vi "XML_EEG_MatLabStringToWaveform.vi"(8 "error in (no error)":errorcluster, 9 "SampleRateHz":dbl, 11 "Hex String in":string) -> (0 "error out":errorcluster, 3 "Waveform out":waveform(dbl))   [LabVIEW 2016, in "XML_EEG_File_Parser.lvlib"]
uses:
  XML_EEG_File_Parser.lvlib
panel:
  # "This VI is a part of BCI Design library, http://www.ru-bci.org \nCopyright © 2020, Sotnikov Peter, All rights reserved. License: GNU GPLv3"
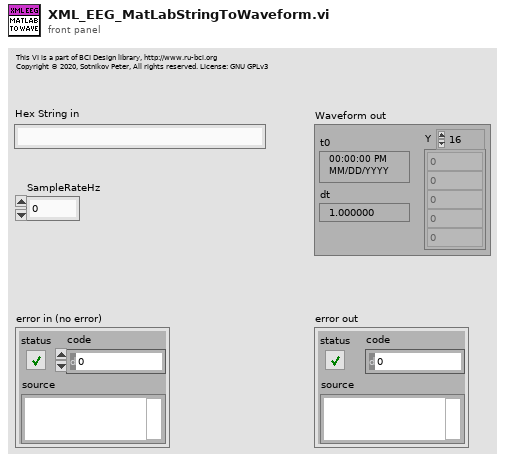
[diagram p1: front panel]
types:
  T1 = enum16{"big-endian, network order", "native, host order", "little-endian"}
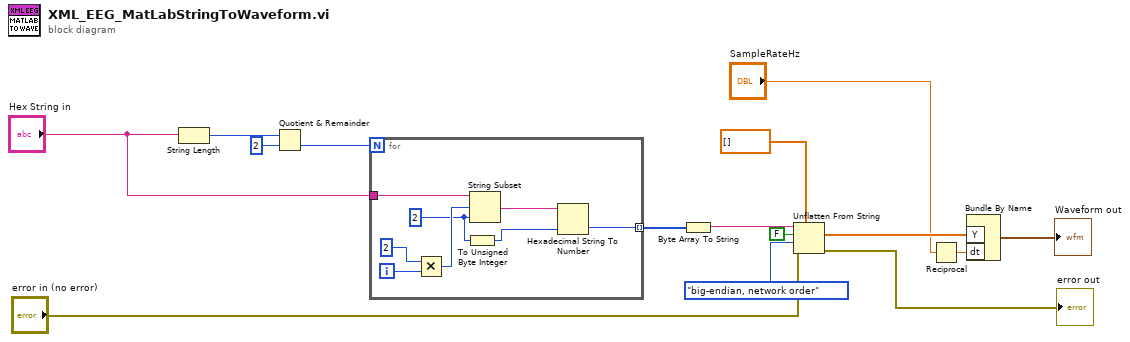
[diagram p0: block diagram]
diagram:
  n1 = String Length(string="Hex String in") -> (length=w15:i32)
  n2 = Quotient & Remainder(x=w15, y=2) -> (floor(x/y)=w13:i32)  [unwired: 1 out]
  n3 = for {
    N: w13 -> [_]
    tunnel: "Hex String in" -> [w23]
    tunnel: [w16] -> w11 mode=indexing
    i -> [w22]
    w18 = 2 ("length (rest)")
    n4 = Multiply(x=2, y=w22) -> (x*y=w20:i32)
    n5 = To Unsigned Byte Integer(number=w18) -> (unsigned 8bit integer=w19:u8)
    n6 = String Subset(string=w23, offset (0)=w20, length (rest)=w18) -> (substring=w17:string)
    n7 = Hexadecimal String To Number(string=w17, default (0uL)=w19) -> (number=w16:u8)  [unwired: 1 in, 1 out]
  }
  n8 = Byte Array To String(unsigned byte array=w11) -> (string=w10:string)
  n9 = Unflatten From String(type=dbl[] [], binary string=w10, data includes array or string size? (T)=FALSE, byte order (0:big-endian, network order)=T1."big-endian, network order", error in (no error)="error in (no error)") -> (value=w3:dbl[], error out=→"error out":errorcluster)  [unwired: 1 out]
  n10 = Reciprocal(x="SampleRateHz") -> (1/x=w2:dbl)
  n11 = Bundle By Name("Y"=w3, "dt"=w2) -> (→"Waveform out":waveform(dbl))  [unwired: 1 in]
